vi "Hasall_extension_numbers_response.vi"(8 "error in (no error)":errorcluster, 11 "OneOfTemplate in":refnum<class "grpc_reflection_v1alpha_ServerReflectionResponse_message_response.lvclass">) -> (0 "error out":errorcluster, 2 "Has Data?":bool, 3 "OneOfTemplate out":refnum<class "grpc_reflection_v1alpha_ServerReflectionResponse_message_response.lvclass">)   [LabVIEW 2019, in "reflection_client.lvlib" / "grpc_reflection_v1alpha_ServerReflectionResponse_message_response.lvclass"]
uses:
  grpc_reflection_v1alpha_ServerReflectionResponse_message_response.lvclass
  grpc_reflection_v1alpha_ServerReflectionResponse_message_response.lvclass/grpc_reflection_v1alpha_ServerReflectionResponse_message_response.ctl
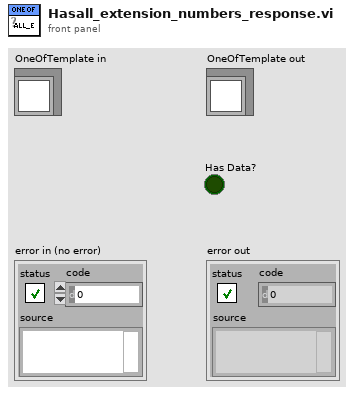
[diagram p1: front panel]
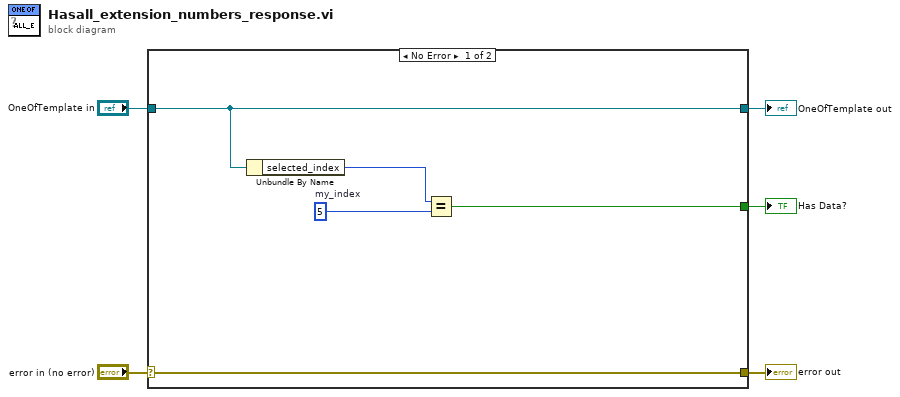
[diagram p0: block diagram]
diagram:
  n1 = case shown="No Error" "error in (no error)" {
    selector: "error in (no error)" -> [w10 w12]
    tunnel: [w10 w12] -> w4
    tunnel: [w9 w11] -> w2
    tunnel: "OneOfTemplate in" -> [w9 w11]
    tunnel: [w6 _] -> w1
    frame No Error {
      w7 = 5  # my_index
      n2 = Unbundle By Name(w9) -> ("selected_index"=w8:i32)
      n3 = Equal?(x=w8, y=w7) -> (x = y?=w6:bool)
    }
    frame Error {
    }
  }
  "error out" <- w4
  "OneOfTemplate out" <- w2
  "Has Data?" <- w1
